vi "M100UtilizationEric.vi"() -> ()   [LabVIEW 2012]
uses:
  <vilib>/Utility/NIReport.llb/NI_report.lvclass
  <vilib>/addons/database/Connection.llb/DB Tools Open Connec (Path).vi
  <vilib>/addons/database/Connection.llb/Conn Execute.vi
  <vilib>/addons/database/Recordset.llb/Rec Fetch Recordset Data (R).vi
  <vilib>/addons/database/Recordset.llb/Rec Destroy - Connection.vi
  <vilib>/Utility/NIReport.llb/Append Text Table to Report (wrap).vi
  <vilib>/addons/database/_DB Variant To Data/Database Variant To Data.xnode
  <vilib>/addons/database/NI_Database_API.lvlib
  <vilib>/Utility/NIReport.llb/Excel/NI_Excel.lvclass
  <vilib>/addons/_office/NI_ReportGenerationToolkit.lvlib
panel:
  out "error out 2":errorcluster
  in  "Table Control":string[][](table)
  out "error out":errorcluster
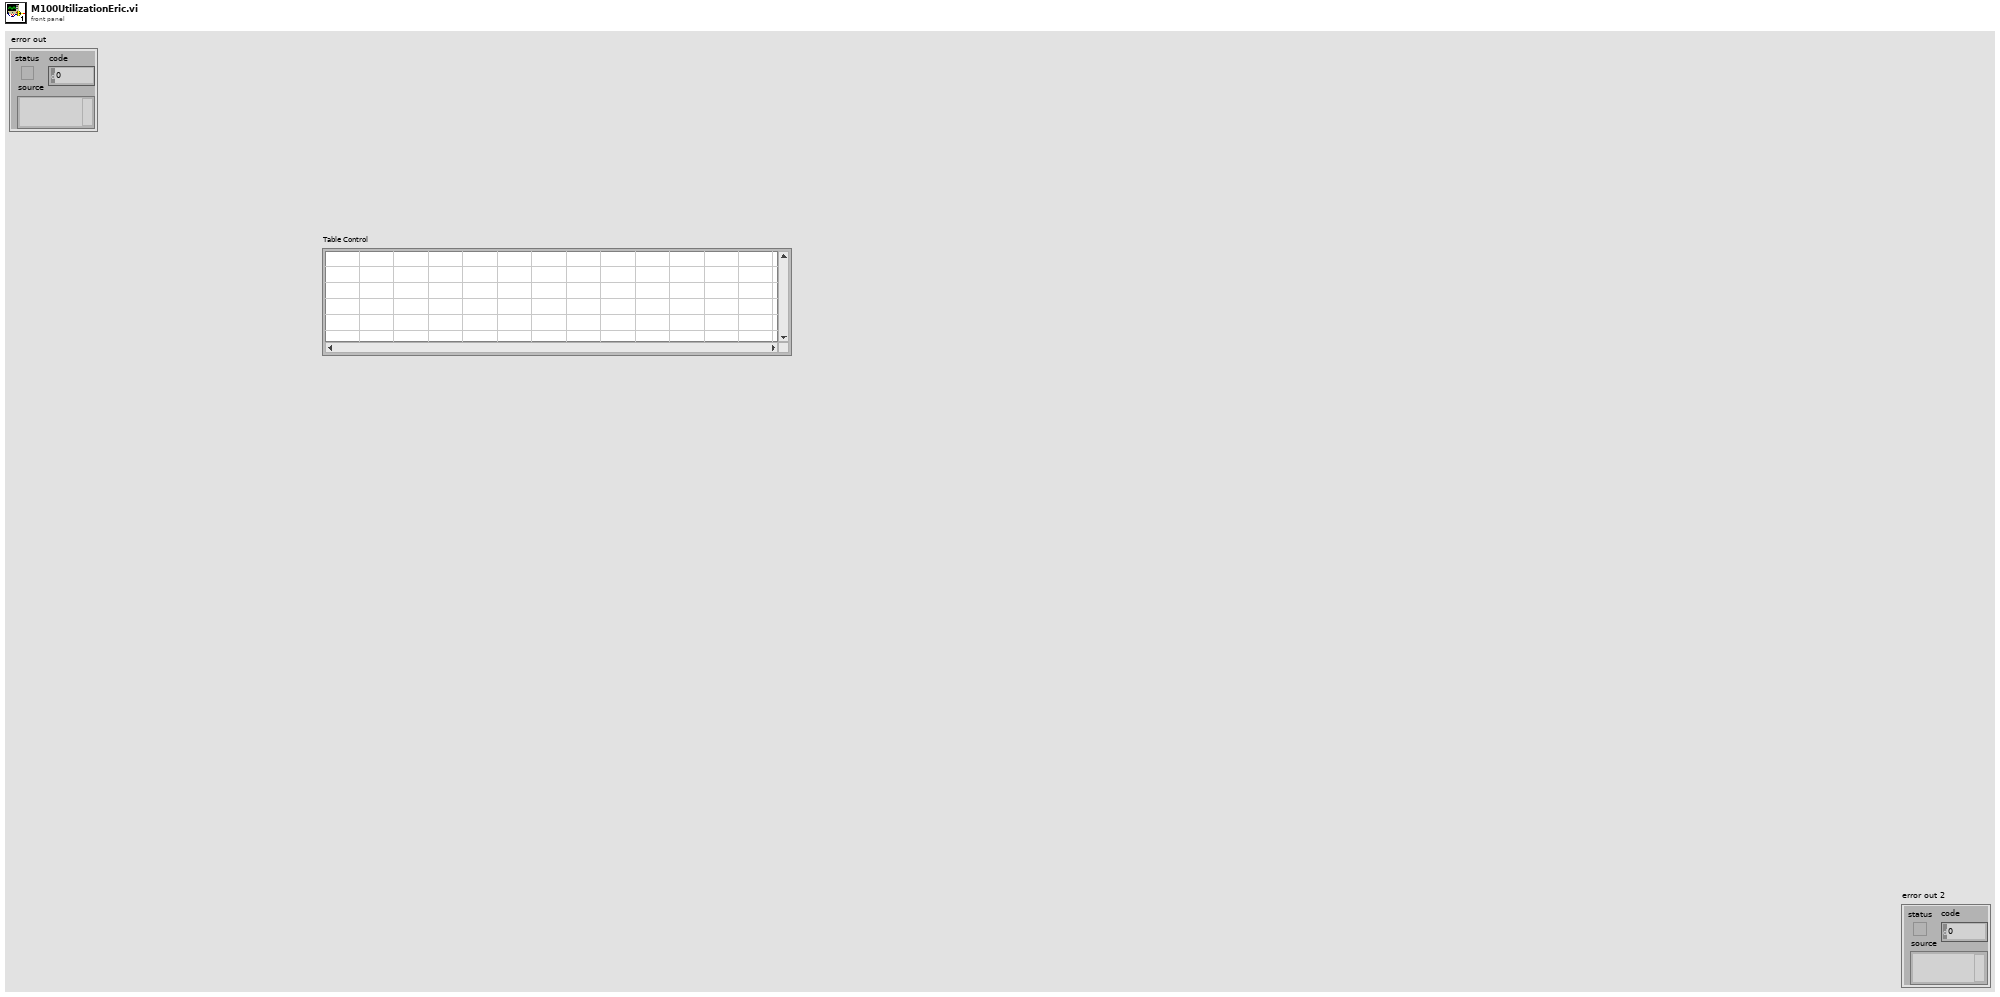
[diagram p1: front panel]
types:
  T1 = typedef "NI_Database_API.lvlib/Conn ObjectReference.ctl" = refnum<k1>
  T2 = typedef "NI_Database_API.lvlib/Rec ObjectReference.ctl" = refnum<k1>
  T3 = enum16{"Standard Report", "HTML", "Word", "Excel"}
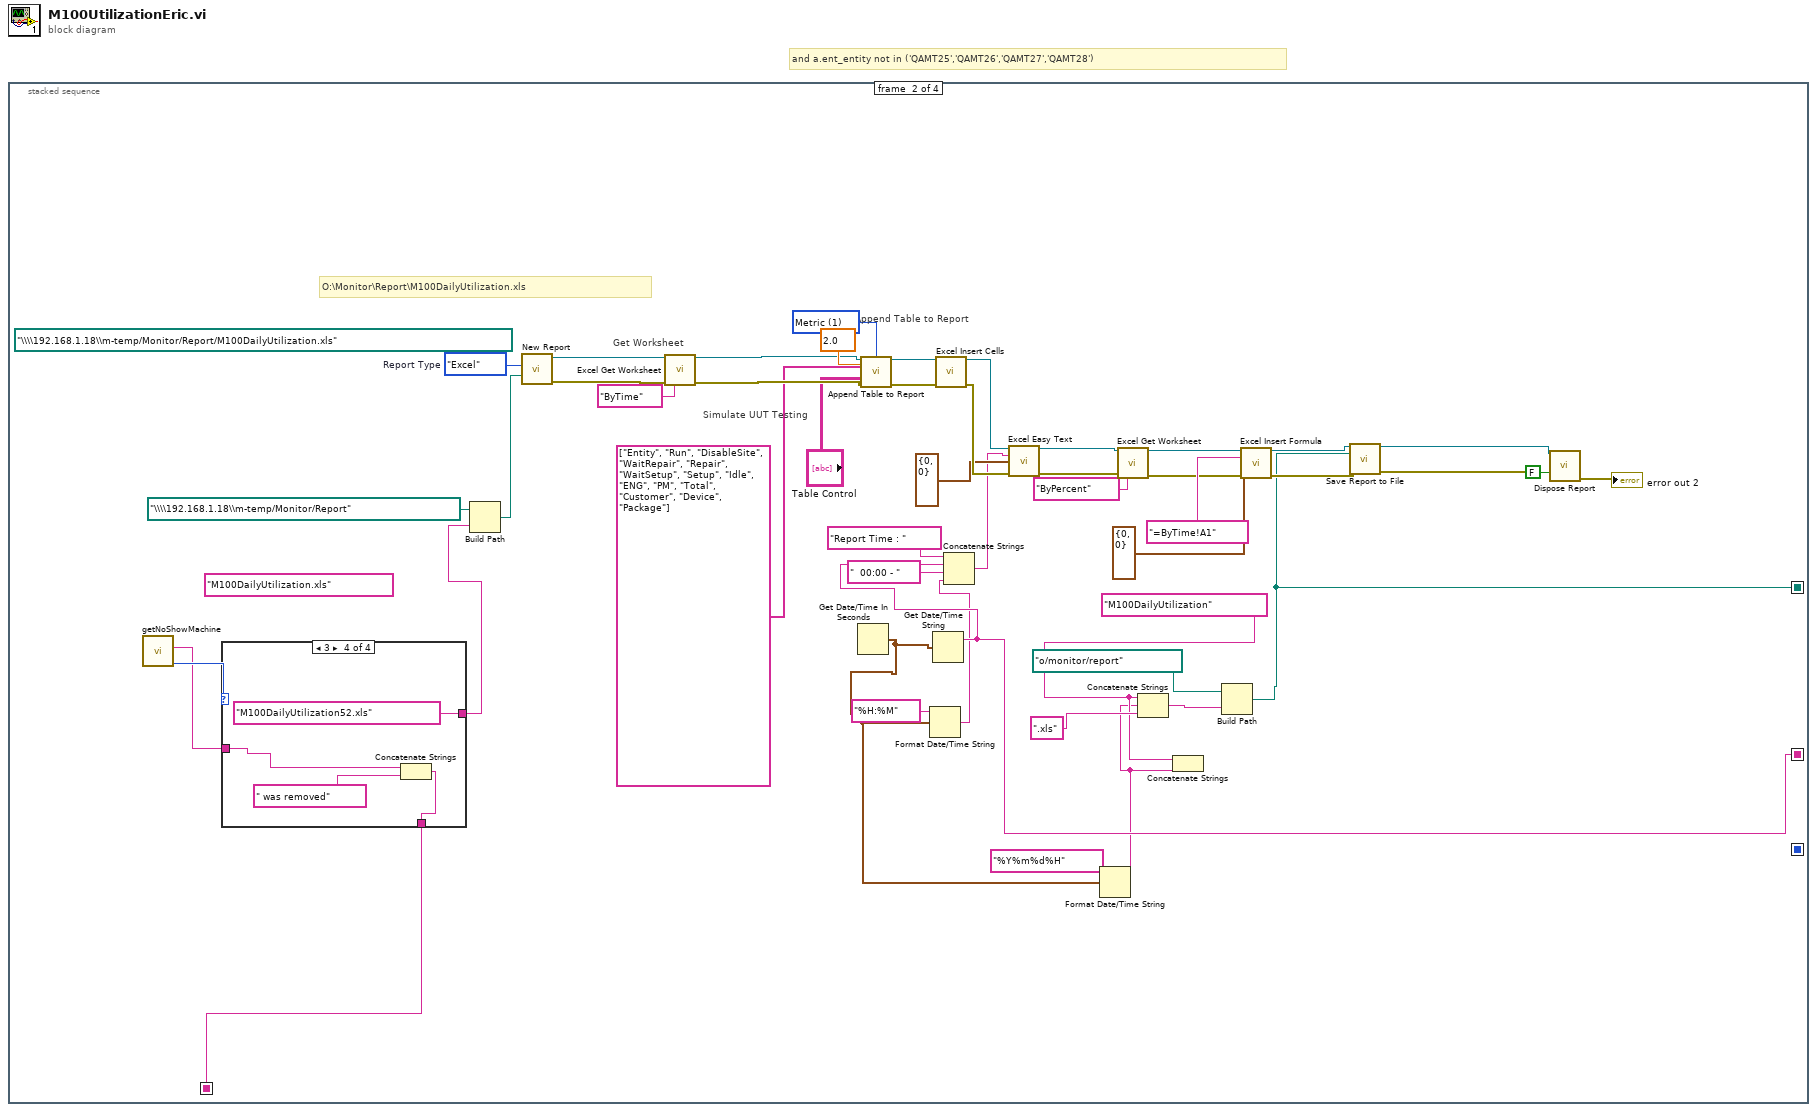
[diagram p0: block diagram]
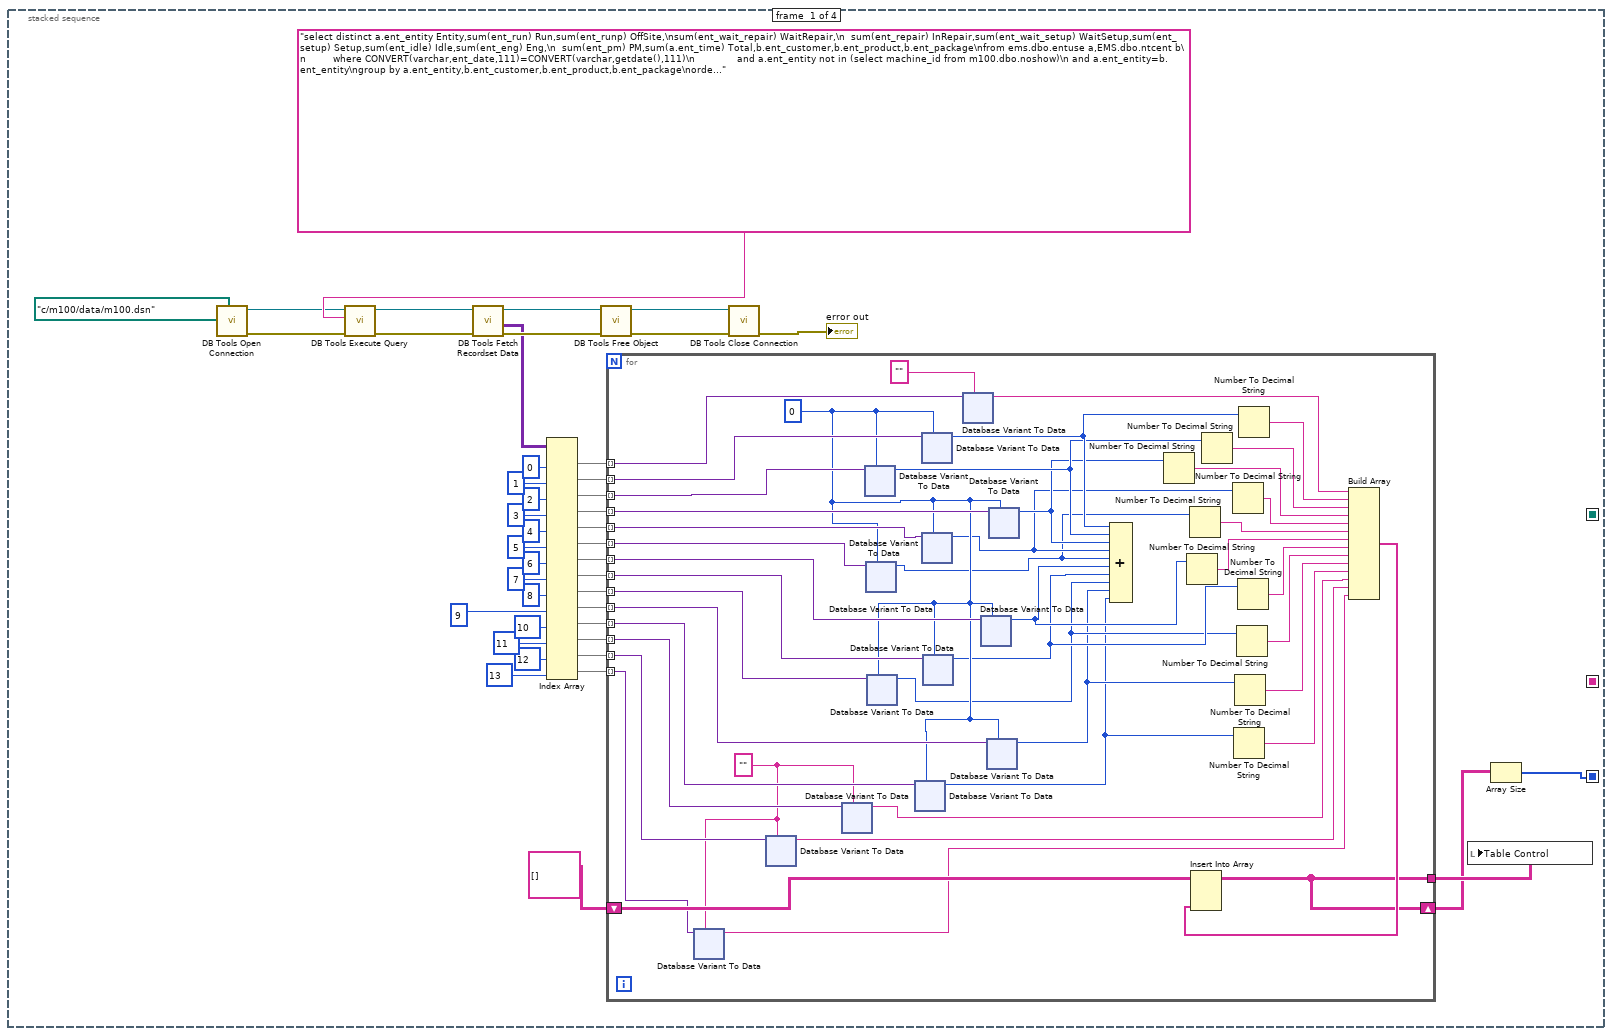
[diagram p2: hidden frame]
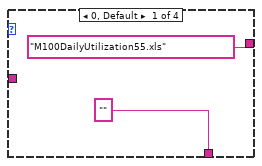
[diagram p3: hidden frame]
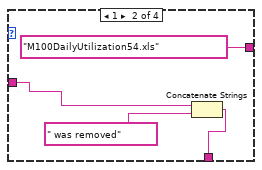
[diagram p4: hidden frame]
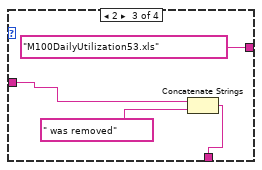
[diagram p5: hidden frame]
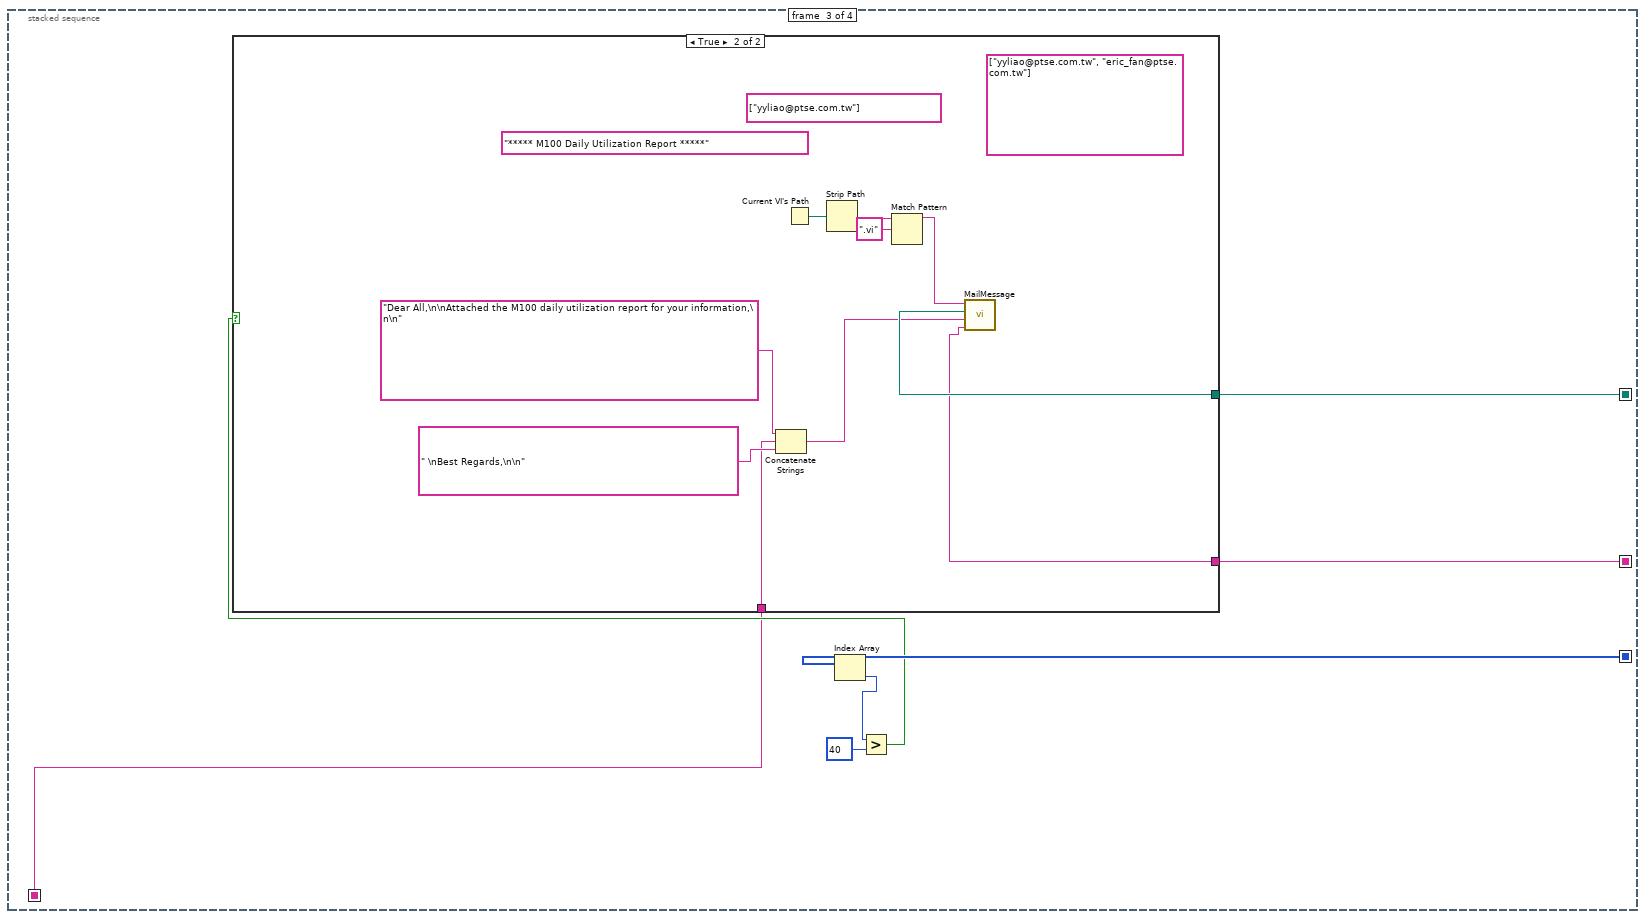
[diagram p6: hidden frame]
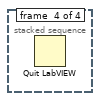
[diagram p8: hidden frame]
diagram:
  # "and a.ent_entity not in ('QAMT25','QAMT26','QAMT27','QAMT28')"
  n1 = stacked-sequence {
    seq-local: [_ w552 _ _] -> [_ _ w605 _]
    seq-local: [_ w551 _ _] -> [_ _ w604 _]
    seq-local: [w7 _ _ _] -> [_ _ w603 _]
    seq-local: [_ w538 _ _] -> [_ _ w599 _]
    frame #0 {
      n2 = call-poly <vilib>:"DB Tools Open Connection.vi"("connection information"=path "c:/m100/data/m100.dsn") -> ("error out"=w38:errorcluster, "connection reference"=w42:T1)  [unwired: 7 in]
      n3 = call-poly <vilib>:"DB Tools Execute Query.vi"("error in (no error)"=w38, "SQL query"="select distinct a.ent_entity Entity,sum(ent_run) Run,sum(ent_runp) OffSite,\nsum(ent_wait_repair) WaitRepair,\n  sum(ent_repair) InRepair,sum(ent_wait_setup) WaitSetup,sum(ent_setup) Setup,sum(ent_idle) Idle,sum(ent_eng) Eng,\n  sum(ent_pm) PM,sum(a.ent_time) Total,b.ent_customer,b.ent_product,b.ent_package\nfrom ems.dbo.entuse a,EMS.dbo.ntcent b\n         where CONVERT(varchar,ent_date,111)=CONVERT(varchar,getdate(),111)\n              and a.ent_entity not in (select machine_id from m100.dbo.noshow)\n and a.ent_entity=b.ent_entity\ngroup by a.ent_entity,b.ent_customer,b.ent_product,b.ent_package\norder by a.ent_entity", "connection reference"=w42) -> ("error out"=w37:errorcluster, "recordset reference"=w41:T2)  [unwired: 5 in]
      n4 = call-poly <vilib>:"DB Tools Fetch Recordset Data.vi"("error in (no error)"=w37, "recordset reference"=w41) -> ("error out"=w36:errorcluster, "recordset data"=w33:variant[][], "recordset reference out"=w40:T2)  [unwired: 3 in]
      n5 = Index Array(array=w33, index (col) #1=0 ("disabled index (col)"), index (col) #2=1 ("index (col)"), index (col) #3=2 ("index (col)"), index (col) #4=3 ("index (col)"), index (col) #5=4 ("index (col)"), index (col) #6=5 ("index (col)"), index (col) #7=6 ("index (col)"), index (col) #8=7 ("index (col)"), index (col) #9=8 ("index (col)"), index (col) #10=9 ("index (col)"), index (col) #11=10 ("index (col)"), index (col) #12=11 ("index (col)"), index (col) #13=12 ("index (col)"), index (col) #14=13 ("index (col)")) -> (element #1=w21:variant[], element #2=w20:variant[], element #3=w19:variant[], element #4=w18:variant[], element #5=w17:variant[], element #6=w16:variant[], element #7=w15:variant[], element #8=w14:variant[], element #9=w13:variant[], element #10=w12:variant[], element #11=w11:variant[], element #12=w4:variant[], element #13=w3:variant[], element #14=w1:variant[])  [unwired: 14 in]
      n6 = call-poly <vilib>:"DB Tools Free Object.vi"("error in (no error)"=w36, "recordset reference"=w40) -> ("error out"=w35:errorcluster, "connection reference"=w39:T1)  [unwired: 8 in]
      n7 = for {
        tunnel: w21 -> [w88] mode=indexing
        tunnel: w20 -> [w87] mode=indexing
        tunnel: w19 -> [w86] mode=indexing
        tunnel: w18 -> [w85] mode=indexing
        tunnel: w17 -> [w84] mode=indexing
        tunnel: w16 -> [w83] mode=indexing
        tunnel: w15 -> [w82] mode=indexing
        tunnel: w14 -> [w81] mode=indexing
        tunnel: w13 -> [w80] mode=indexing
        tunnel: w12 -> [w79] mode=indexing
        tunnel: w11 -> [w78] mode=indexing
        tunnel: [w53] -> w9
        shift-right: [w53] -> w8
        shift-left: string[][] [] ("array") -> [w52]
        tunnel: w4 -> [w51] mode=indexing
        tunnel: w3 -> [w50] mode=indexing
        tunnel: w1 -> [w47] mode=indexing
        w46 = ""
        w76 = 0
        n8 = xnode "Database Variant To Data"("database variant"=w47, "type"=w46) -> ("data"=w45:string)  [unwired: 1 in, 1 out]
        n9 = xnode "Database Variant To Data"("database variant"=w50, "type"=w46) -> ("data"=w48:string)  [unwired: 1 in, 1 out]
        n10 = xnode "Database Variant To Data"("database variant"=w51, "type"=w46) -> ("data"=w49:string)  [unwired: 1 in, 1 out]
        n11 = xnode "Database Variant To Data"("database variant"=w86, "type"=w76) -> ("data"=w72:i32)  [unwired: 1 in, 1 out]
        n12 = xnode "Database Variant To Data"("database variant"=w83, "type"=w76) -> ("data"=w66:i32)  [unwired: 1 in, 1 out]
        n13 = xnode "Database Variant To Data"("database variant"=w80, "type"=w76) -> ("data"=w60:i32)  [unwired: 1 in, 1 out]
        n14 = xnode "Database Variant To Data"("database variant"=w78, "type"=w76) -> ("data"=w56:i32)  [unwired: 1 in, 1 out]
        n15 = xnode "Database Variant To Data"("database variant"=w87, "type"=w76) -> ("data"=w75:i32)  [unwired: 1 in, 1 out]
        n16 = xnode "Database Variant To Data"("database variant"=w84, "type"=w76) -> ("data"=w68:i32)  [unwired: 1 in, 1 out]
        n17 = xnode "Database Variant To Data"("database variant"=w81, "type"=w76) -> ("data"=w62:i32)  [unwired: 1 in, 1 out]
        n18 = xnode "Database Variant To Data"("database variant"=w88, "type"="") -> ("data"=w74:string)  [unwired: 1 in, 1 out]
        n19 = xnode "Database Variant To Data"("database variant"=w82, "type"=w76) -> ("data"=w64:i32)  [unwired: 1 in, 1 out]
        n20 = xnode "Database Variant To Data"("database variant"=w79, "type"=w76) -> ("data"=w58:i32)  [unwired: 1 in, 1 out]
        n21 = xnode "Database Variant To Data"("database variant"=w85, "type"=w76) -> ("data"=w70:i32)  [unwired: 1 in, 1 out]
        n22 = Compound Arithmetic op=ADD(w75, w72, w70, w68, w66, w64, w62, w60, w58, w56) -> ()  [unwired: 1 out]
        n23 = Number To Decimal String(number=w70) -> (decimal integer string=w69:string)  [unwired: 1 in]
        n24 = Number To Decimal String(number=w64) -> (decimal integer string=w63:string)  [unwired: 1 in]
        n25 = Number To Decimal String(number=w66) -> (decimal integer string=w65:string)  [unwired: 1 in]
        n26 = Number To Decimal String(number=w72) -> (decimal integer string=w71:string)  [unwired: 1 in]
        n27 = Number To Decimal String(number=w68) -> (decimal integer string=w67:string)  [unwired: 1 in]
        n28 = Number To Decimal String(number=w56) -> (decimal integer string=w55:string)  [unwired: 1 in]
        n29 = Number To Decimal String(number=w58) -> (decimal integer string=w57:string)  [unwired: 1 in]
        n30 = Number To Decimal String(number=w60) -> (decimal integer string=w59:string)  [unwired: 1 in]
        n31 = Number To Decimal String(number=w62) -> (decimal integer string=w61:string)  [unwired: 1 in]
        n32 = Number To Decimal String(number=w75) -> (decimal integer string=w73:string)  [unwired: 1 in]
        n33 = Build Array(w74, w73, w71, w69, w67, w65, w63, w61, w59, w57, w55, w49, w48, w45) -> (w54:string[])
        n34 = Insert Into Array(array=w52, new element=w54) -> (w53:string[][])  [unwired: 2 in]
      }
      n35 = call <vilib>:"DB Tools Close Connection.vi"("error in (no error)"=w35, "connection reference"=w39) -> ("error out"=→"error out":errorcluster)  [unwired: 5 in]
      n36 = local write "Table Control"(w9) -> ()
      n37 = Array Size(array=w8) -> (size(s)=w7:i32[])
    }
    frame #1 {
      (unwired) path "\\\\192.168.1.18\\m-temp/Monitor/Report/M100DailyUtilization.xls" ("template (empty)")
      (unwired) "M100DailyUtilization.xls" ("name or relative path")
      w549 = u16 1 items=["US", "Metric", "Default"] ("measurement system")
      w553 = "M100DailyUtilization"
      w584 = T3."Excel"  # Report Type
      # "O:\\Monitor\\Report\\M100DailyUtilization.xls"
      # "Simulate UUT Testing"
      # "Append Table to Report"
      # "Get Worksheet"
      n38 = call "getNoShowMachine.vi"() -> ("rows"=w540:i32, "Machine"=w537:string)  [unwired: 10 in]
      n39 = case shown="3" w540 {
        tunnel: ["M100DailyUtilization55.xls" ("name or relative path") "M100DailyUtilization54.xls" ("name or relative path") "M100DailyUtilization53.xls" ("name or relative path") "M100DailyUtilization52.xls" ("name or relative path")] -> w539
        tunnel: ["" w587 w591 w595] -> w538
        tunnel: w537 -> [_ w589 w592 w596]
        frame 0, Default {
        }
        frame 1 {
          n40 = Concatenate Strings(w589, " was removed" ("string")) -> (w587:string)
        }
        frame 2 {
          n41 = Concatenate Strings(w592, " was removed" ("string")) -> (w591:string)
        }
        frame 3 {
          n42 = Concatenate Strings(w596, " was removed" ("string")) -> (w595:string)
        }
      }
      n43 = Build Path(base path=path "\\\\192.168.1.18\\m-temp/Monitor/Report", name or relative path=w539) -> (appended path=w541:path)
      n44 = call <vilib>:"New Report.vi"("report type"=w584, "template (empty)"=w541) -> ("report out"=w580:refnum<class "NI_report.lvclass">, "error out"=w579:errorcluster)  [unwired: 12 in]
      n45 = call <vilib>:"Excel Get Worksheet.vi"("report in"=w580, "error in (no error)"=w579, "name (\"\")"="ByTime" ("name (\"\")")) -> ("report out"=w569:refnum<class "NI_report.lvclass">, "error out"=w568:errorcluster)  [unwired: 11 in]
      n46 = Get Date/Time In Seconds() -> (seconds since 1Jan1904=w545:timestamp)
      n47 = call-poly <vilib>:"Append Table to Report.vi"("report in"=w569, "column width (1)"=2.0, "measurement system"=w549, "column headers"=string[] ["Entity", "Run", "DisableSite", "WaitRepair", "Repair", "WaitSetup", "Setup", "Idle", "ENG", "PM", "Total", "Customer", "Device", "Package"] ("row headers"), "text data"="Table Control", "error in (no error)"=w568) -> ("report out"=w582:refnum<class "NI_report.lvclass">, "error out"=w581:errorcluster)  [unwired: 6 in, 2 out]
      n48 = Format Date/Time String(time format string (%c)="%H:%M", seconds (now)=w545) -> (date/time string=w543:string)  [unwired: 1 in]
      n49 = Get Date/Time String(seconds (now)=w545) -> (date string=w551:string)  [unwired: 2 in, 1 out]
      n50 = call <vilib>:"Excel Insert Cells.vi"("report in"=w582, "error in (no error)"=w581) -> ("report out"=w576:refnum<class "NI_report.lvclass">, "error out"=w575:errorcluster)  [unwired: 12 in]
      n51 = Concatenate Strings("Report Time : " ("string"), w551, "  00:00 - " ("string"), w543) -> (w572:string)
      n52 = call <vilib>:"Excel Easy Text.vi"("report in"=w576, "text"=w572, "start (-1, -1)"=cluster{"row":i32, "column":i32} {"row"=0, "column"=0} ("end (-1, -1)"), "error in (no error)"=w575) -> ("report out"=w565:refnum<class "NI_report.lvclass">, "error out"=w564:errorcluster)  [unwired: 7 in, 3 out]
      n53 = Format Date/Time String(time format string (%c)="%Y%m%d%H", seconds (now)=w545) -> (date/time string=w547:string)  [unwired: 1 in]
      n54 = call <vilib>:"Excel Get Worksheet.vi"("report in"=w565, "error in (no error)"=w564, "name (\"\")"="ByPercent" ("name (\"\")")) -> ("report out"=w560:refnum<class "NI_report.lvclass">, "error out"=w559:errorcluster)  [unwired: 11 in]
      n55 = Concatenate Strings(w553, w547, ".xls" ("string")) -> (w554:string)
      n56 = Concatenate Strings(w553, w547) -> ()  [unwired: 1 out]
      n57 = Build Path(base path=path "o:/monitor/report", name or relative path=w554) -> (appended path=w552:path)
      n58 = call <vilib>:"Excel Insert Formula.vi"("report in"=w560, "formula"="=ByTime!A1", "start (0, 0)"=cluster{"row":i32, "column":i32} {"row"=0, "column"=0}, "error in (no error)"=w559) -> ("report out"=w558:refnum<class "NI_report.lvclass">, "error out"=w557:errorcluster)  [unwired: 10 in]
      n59 = call-dynamic "Save Report to File.vi"("report in"=w558, "report file path"=w552, "error in (no error)"=w557) -> ("report out"=w571:refnum<class "NI_report.lvclass">, "error out"=w570:errorcluster)  [unwired: 11 in]
      n60 = call-dynamic "Dispose Report.vi"("report in"=w571, "save changes? (F)"=FALSE, "error in (no error)"=w570) -> ("error out"=→"error out 2":errorcluster)  [unwired: 12 in]
    }
    frame #2 {
      n61 = Index Array(array=w603) -> (element=w602:i32)  [unwired: 1 in]
      n62 = Greater?(x=w602, y=40) -> (0:w600:bool)
      n63 = case shown="True" w600 {
        tunnel: w605 -> [_ w611]
        tunnel: w604 -> [_ w610]
        tunnel: w599 -> [_ w606]
        frame False {
        }
        frame True {
          (unwired) string[] ["yyliao@ptse.com.tw", "eric_fan@ptse.com.tw"] ("recipients")
          (unwired) "***** M100 Daily Utilization Report *****" ("subject ([No Subject])")
          (unwired) string[] ["yyliao@ptse.com.tw"] ("recipients")
          n64 = Concatenate Strings("Dear All,\n\nAttached the M100 daily utilization report for your information,\n\n" ("message"), w606, " \nBest Regards,\n\n" ("message")) -> (w608:string)
          n65 = Current VI's Path() -> (path=w615:path)
          n66 = Strip Path(path=w615) -> (name=w614:string)  [unwired: 1 out]
          n67 = Match Pattern(string=w614, regular expression=".vi") -> (before substring=w612:string)  [unwired: 1 in, 3 out]
          n68 = call "MailMessage.vi"("AddSubject"=w610, "message"=w608, "file path"=w611, "program"=w612) -> ()  [unwired: 8 in]
        }
      }
    }
    frame #3 {
      n69 = Quit LabVIEW() -> ()  [unwired: 1 in]
    }
  }
